vi "GetVideoOptionsCodes.vi"(8 "error in (no error)":errorcluster, 11 "Camera in":refnum<class "Camera.lvclass">) -> (0 "error out":errorcluster, 2 "VideoOptionsCodes":T1 {"ImageTypeCodesList"."Code" format="%.0x"; "VideoResolutionCodesList"."Code" format="%.0x"; "FrameRateCodesList"."Code" format="%.0x"}, 3 "Camera out":refnum<class "Camera.lvclass">)   [LabVIEW 2020, in "CameraUSB.lvlib" / "Camera.lvclass"]
uses:
  Camera.lvclass
  ICamera/TypeDef/VideoOptionsCodes.ctl
  Camera.lvclass/Camera.ctl
  ICamera/TypeDef/ICamera_typedef.lvlib
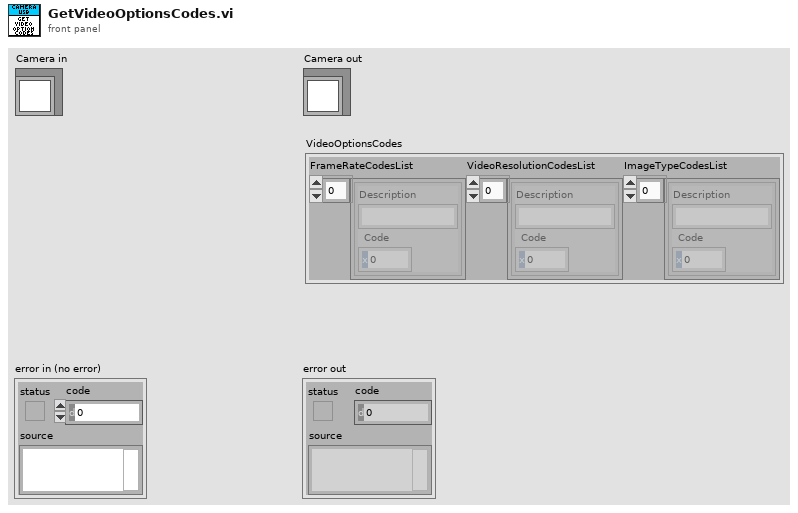
[diagram p1: front panel]
types:
  T1 = typedef "ICamera_typedef.lvlib/VideoOptionsCodes.ctl" = cluster{"FrameRateCodesList":cluster{"Description":string, "Code":u8}[], "VideoResolutionCodesList":cluster{"Description":string, "Code":u8}[], "ImageTypeCodesList":cluster{"Description":string, "Code":u8}[]}
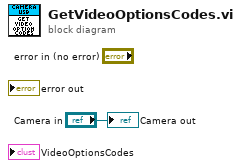
[diagram p0: block diagram]
diagram:
  "Camera out" <- "Camera in"
